vi "Teleop.vi.LOCAL.vi"(9 "Match Info":T1={"Autonomous Elapsed Seconds"=0.0, "TeleOp Elapsed Seconds"=0.0, "Disabled Elapsed Seconds"=0.0, "Visited Autonomous"=FALSE, "Visited TeleOp"=FALSE, "Visited Disabled"=FALSE, "Autonomous Settings"={"Autonomous Style"=enum."Independent", "VI Refnum"=refnum}}, 11 "Call Context":T2) -> (0 "output cluster":cluster{"output":dbl, "output":dbl}, 1 "Encoder Rate":cluster{"Rate":dbl, "Rate":dbl})   [LabVIEW 2013]
doc: "This VI is called for each TeleOp packet received from the DS where the robot is not disabled. It is often used to read from the joysticks and update I/O or to update setpoints for timed control loops. It should complete and return within 20 milliseconds or it may miss DS packets."
uses:
  <vilib>/Rock Robotics/WPI/DriverStation/WPI_DriverStationDerivedRobotMode.ctl
  <vilib>/Rock Robotics/WPI/DriverStation/WPI_DriverStationMatch Info.ctl
  Robot Global Data.vi
  Global.vi
  <vilib>/Rock Robotics/WPI/RobotDrive/WPI_RobotDriveGetSetRefNum.vi
panel:
  in  "D":dbl
  in  "I":dbl=0.01
  in  "P":dbl=1.3
  out "error out":errorcluster
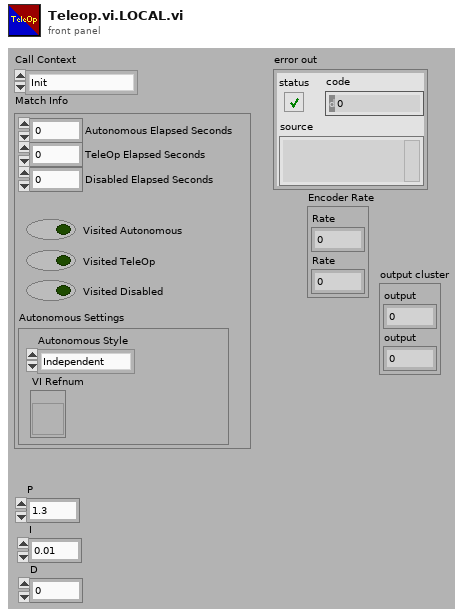
[diagram p1: front panel]
types:
  T1 = typedef "WPI_DriverStationMatch Info.ctl" = cluster{"Autonomous Elapsed Seconds":dbl, "TeleOp Elapsed Seconds":dbl, "Disabled Elapsed Seconds":dbl, "Visited Autonomous":bool, "Visited TeleOp":bool, "Visited Disabled":bool, "Autonomous Settings":cluster{"Autonomous Style":enum16{"Iterative", "Independent"}, "VI Refnum":refnum<vi>}}
  T2 = typedef "WPI_DriverStationDerivedRobotMode.ctl" = enum16{"Init", "Execute", "Stop"}
  T3 = typedef "WPI_RobotDriveDevRef.ctl" = cluster{"DevStatus":errorcluster, "Motors[]":T4[], "Square Inputs":bool, "Max Output":dbl, "Isochronous":bool}
  T4 = typedef "WPI_MotorControlDeviceRef.ctl" = cluster{"DeviceStatus":errorcluster, "Type":enum16{"PWM", "CAN"}, "PWM":cluster{"Digital Module":T5, "PWM Channel":T6, "DeadBand":T7}, "CAN":cluster{"Device Number":u8, "Control Mode":T8, "Semaphore":T9, "Max Vout":dbl}, "Invert":bool, "TransformRef":T10, "InvTransformRef":T10}
  T5 = typedef "FPGA_TypedefDigitalModule.ctl" = enum16{"Digital Module 1", "Digital Module 2"}
  T6 = typedef "FPGA_DIOPWMChannel.ctl" = enum8{"PWM 1", "PWM 2", "PWM 3", "PWM 4", "PWM 5", "PWM 6", "PWM 7", "PWM 8", "PWM 9", "PWM 10", "Invalid"}
  T7 = typedef "WPI_PWMDeadband.ctl" = cluster{"Name":string, "maxPositivePwm":i32, "minPositivePwm":i32, "centerPwm":i32, "maxNegativePwm":i32, "minNegativePwm":i32, "angularRange":u16}
  T8 = typedef "WPI_CANJaguar_ControlMode.ctl" = enum8{"Percent VBus", "Current", "Speed", "Position", "Voltage"}
  T9 = typedef "Semaphore RefNum" = refnum<k1>
  T10 = typedef "WPI_PWMTransform_ConPane.ctl" = refnum<vi>
  T11 = cluster{"X":bool, "A":bool, "B":bool, "Y":bool, "LB":bool, "RB":bool, "LT":bool, "RT":bool, "Back":bool, "Start":bool, "LC":bool, "RC":bool}
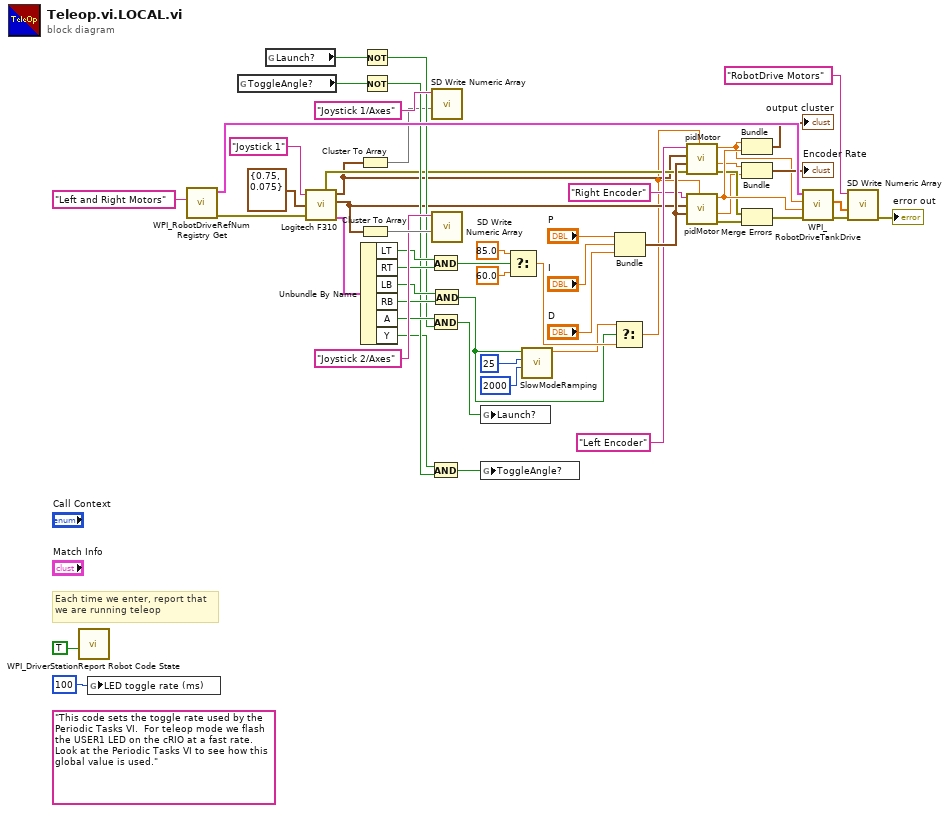
[diagram p0: block diagram]
diagram:
  (unwired) "This code sets the toggle rate used by the Periodic Tasks VI.  For teleop mode we flash the USER1 LED on the cRIO at a fast rate.  Look at the Periodic Tasks VI to see how this global value is used."
  # "Each time we enter, report that\nwe are running teleop"
  n1 = call <vilib>:"WPI_DriverStationReport Robot Code State.vi"("TeleOp"=TRUE ("Autonomous")) -> ()  [unwired: 10 in, 1 out]
  n2 = global write "Robot Global Data.vi" "LED toggle rate (ms)"(u32 100 ("LED ms toggle rate")) -> ()
  n3 = call <vilib>:"WPI_RobotDriveRefNum Registry Get.vi"("refnum name"="Left and Right Motors") -> ("error out"=w42:errorcluster, "RobotDriveDevRef"=w52:T3)  [unwired: 9 in]
  n4 = global read "Global.vi" "ToggleAngle?"() -> (w22:bool)
  n5 = global read "Global.vi" "Launch?"() -> (w25:bool)
  n6 = call "Logitech F310.vi"("error in (no error)"=w42, "Deadzone Scale Cluster"=cluster{"Scale":dbl, "Deadzone":dbl} {"Scale"=0.75, "Deadzone"=0.075}, "refnum name"="Joystick 1") -> ("Buttons"=w36:T11, "Right Stick"=w4:cluster{"X":dbl, "Y":dbl}, "error out"=w8:errorcluster, "Left Stick"=w5:cluster{"X":dbl, "Y":dbl})  [unwired: 2 out]
  n7 = Cluster To Array(cluster=w5) -> (array=w9:dbl[])
  n8 = Cluster To Array(cluster=w4) -> (array=w39:dbl[])
  n9 = Unbundle By Name(w36) -> ("LT"=w35:bool, "RT"=w34:bool, "LB"=w29:bool, "RB"=w28:bool, "A"=w27:bool, "Y"=w20:bool)
  n10 = Not(x=w25) -> (.not. x?=w24:bool)
  n11 = Not(x=w22) -> (.not. x?=w21:bool)
  n12 = And(x=w35, y=w34) -> (x .and. y?=w33:bool)
  n13 = And(x=w27, y=w24) -> (x .and. y?=w26:bool)
  n14 = And(x=w20, y=w21) -> (x .and. y?=w23:bool)
  n15 = call <vilib>:"SD Write Numeric Array.vi"("Numeric Array"=w9, "Name"="Joystick 1/Axes") -> ()  [unwired: 8 in, 2 out]
  n16 = call <vilib>:"SD Write Numeric Array.vi"("Numeric Array"=w39, "Name"="Joystick 2/Axes") -> ()  [unwired: 8 in, 2 out]
  n17 = And(x=w29, y=w28) -> (x .and. y?=w18:bool)
  n18 = global write "Global.vi" "Launch?"(w26) -> ()
  n19 = global write "Global.vi" "ToggleAngle?"(w23) -> ()
  n20 = Select(t=85.0, s=w33, f=60.0 ("x")) -> (s? t:f=w32:dbl)
  n21 = call "SlowModeRamping.vi"("Ramp Time (ms)"=u32 2000, "Goal"=25, "SlowMode?"=w18) -> ("Multiplier"=w15:dbl)  [unwired: 8 in]
  n22 = Select(t=w15, s=w18, f=w32) -> (s? t:f=w1:dbl)
  n23 = Bundle("P"="P", "I"="I", "D"="D") -> (w12:cluster{"P":dbl, "I":dbl, "D":dbl})  [unwired: 1 in]
  n24 = call "pidMotor.vi"("Multiplier"=w1, "error in (no error)"=w8, "PID gains"=w12, "Joystic  cluster"=w5, "Encoder"="Left Encoder" ("refnum name")) -> ("error out"=w7:errorcluster, "Rate"=w3:dbl, "output"=w13:dbl)  [unwired: 4 in]
  n25 = call "pidMotor.vi"("Multiplier"=w1, "PID gains"=w12, "Joystic  cluster"=w4, "Encoder"="Right Encoder" ("refnum name")) -> ("error out"=w6:errorcluster, "Rate"=w2:dbl, "output"=w14:dbl)  [unwired: 5 in]
  n26 = Bundle("output"=w13, "output"=w14) -> (→"output cluster":cluster{"output":dbl, "output":dbl})  [unwired: 1 in]
  n27 = Bundle("Rate"=w3, "Rate"=w2) -> (→"Encoder Rate":cluster{"Rate":dbl, "Rate":dbl})  [unwired: 1 in]
  n28 = Merge Errors(w7, w6) -> (w44:errorcluster)
  n29 = call <vilib>:"WPI_RobotDriveTankDrive.vi"("error in (no error)"=w44, "Right axis value"=w14, "Left axis value"=w13, "RobotDriveDevRef"=w52) -> ("error out"=w50:errorcluster, "Motor Values"=w51:dbl[])  [unwired: 5 in, 1 out]
  n30 = call <vilib>:"SD Write Numeric Array.vi"("error in"=w50, "Numeric Array"=w51, "Name"="RobotDrive Motors") -> ("error out"=→"error out":errorcluster)  [unwired: 7 in, 1 out]
